vi "[Global] CoordTemp.vi"() -> ()   [LabVIEW 2015]
panel:
  out "CoordTempArray":string[](array[string])
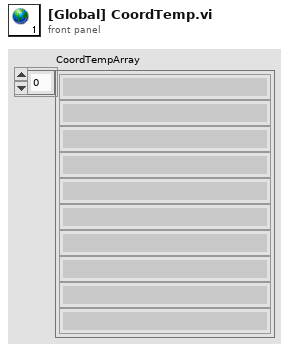
[diagram p1: front panel]
diagram:
